vi "Get Instrument Path.vi"(11 "VI Name":path) -> (2 "VI Name":string, 3 "Instrument Path":path)   [LabVIEW 2021]
doc: "VI to get (or translate) correct path to an instrument for any platform\nScott Hannahs <sth@magnet.fsu.edu>"
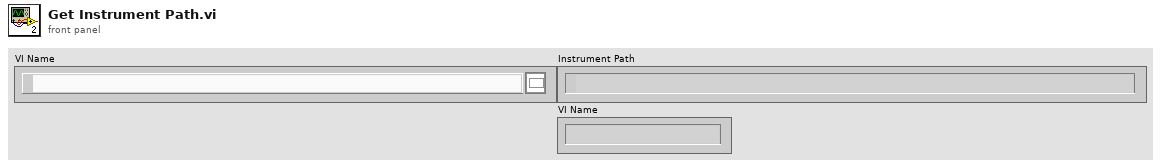
[diagram p1: front panel]
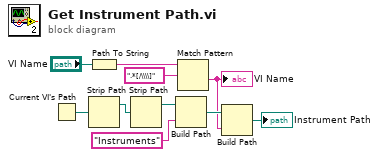
[diagram p0: block diagram]
diagram:
  n1 = Current VI's Path() -> (path=w10:path)
  n2 = Path To String(path="VI Name") -> (string=w1:string)
  n3 = Strip Path(path=w10) -> (stripped path=w9:path)  [unwired: 1 out]
  n4 = Strip Path(path=w9) -> (stripped path=w2:path)  [unwired: 1 out]
  n5 = Build Path(base path=w2, name or relative path="Instruments") -> (appended path=w7:path)
  n6 = Match Pattern(string=w1, regular expression=".*[/\\\\]") -> (after substring=w3:string)  [unwired: 1 in, 3 out]
  "VI Name" <- w3
  n7 = Build Path(base path=w7, name or relative path=w3) -> (appended path=→"Instrument Path":path)
